vi "LVClass_CameraSet Set Parameter StringValue.vi"(0 "CameraSet.lvclass":refnum<class "CameraSet.lvclass">, 5 "parameter name":string, 7 "Value":string, 11 "error in (no error)":errorcluster) -> (4 "CameraSet.lvclass":refnum<class "CameraSet.lvclass">, 15 "error out":errorcluster)   [LabVIEW 2020, in "CameraSet.lvclass"]
doc: "Camera parameter value setter for parameter of type string.\n\n<B>camera_setIn</B> : CameraSet object.\n<B>camera_setOut</B> : CameraSet object.\n<B>parameter_name</B> : Parameter name.\n<B>value</B> : Parameter value."
uses:
  CameraSet.lvclass
  CameraSet.lvclass/CameraSet.ctl
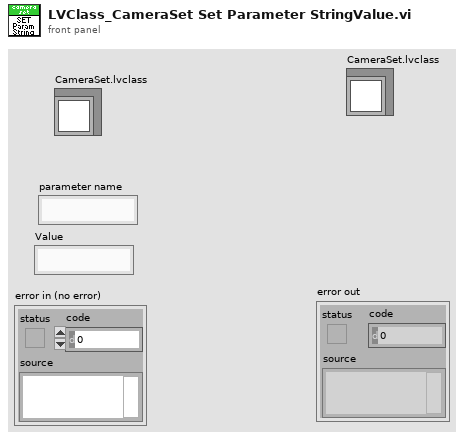
[diagram p1: front panel]
types:
  T1 = typedef "ClassID.ctl" = i64
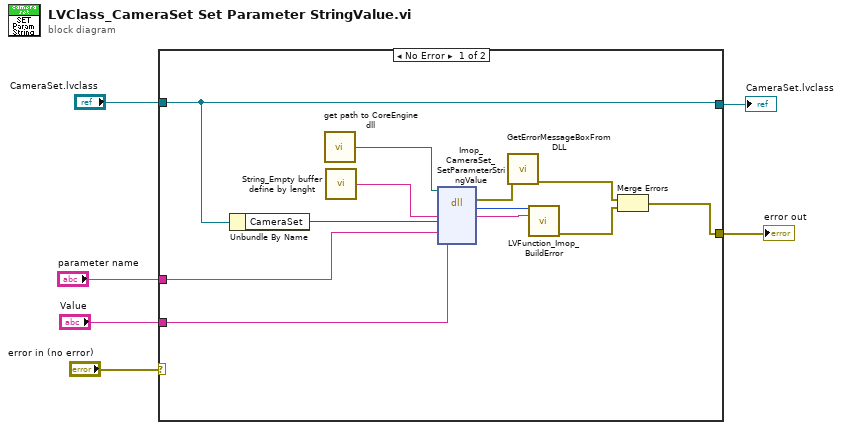
[diagram p0: block diagram]
diagram:
  n1 = case shown="No Error" "error in (no error)" {
    selector: "error in (no error)" -> [_ w19]
    tunnel: "CameraSet.lvclass" -> [w14 w20]
    tunnel: [w14 w20] -> w4
    tunnel: [w10 w19] -> w3
    tunnel: "Value" -> [w9 _]
    tunnel: "parameter name" -> [w7 _]
    frame No Error {
      n2 = Unbundle By Name(w14) -> ("CameraSet"=w13:T1)
      n3 = call "get path to CoreEngine dll.vi"() -> ("path to c_interface_vc100.dll"=w16:path)  [unwired: 12 in, 3 out]
      n4 = call "String_Empty buffer define by lenght.vi"() -> ("Empty buffer"=w8:string)  [unwired: 1 in]
      n5 = dll-call lib="D:/SOFTware/HASO_v3/SVN_trunk/ImOpCoreEngine4_LV2011/DLLs/c_interface_vc100.dll" fn="Imop_CameraSet_SetParameterStringValue"(path in=w16, "message"=w8, "objet"=w13, "parameter name"=w7, "Name"=w9) -> (error out=w15:errorcluster, "return type"=w18:i32, "message"=w17:string)  [unwired: 5 in, 1 out]
      n6 = call "GetErrorMessageBoxFromDLL.vi"("error IN"=w15) -> ("error OUT"=w12:errorcluster)  [unwired: 10 in]
      n7 = call "LVFunction_Imop_BuildError.vi"("code"=w18, "String to Prepend to source (\"\")"=w17) -> ("error out"=w11:errorcluster)  [unwired: 13 in]
      n8 = Merge Errors(w12, w11) -> (w10:errorcluster)
    }
    frame Error {
    }
  }
  "CameraSet.lvclass" <- w4
  "error out" <- w3
